vi "Switch Control.vi"(8 "error in (no error)":errorcluster, 11 "On/Off":bool) -> (0 "error out":errorcluster)   [LabVIEW 2014]
doc: "Turns the Switch on or off. Also turns the LED on or off to notify the user which state the switch is in."
uses:
  Controls/Switch Type.ctl
  <vilib>/myRIO/Instrument Drivers/Onboard IO/DIO/vis/Write.vi
  <vilib>/myRIO/Instrument Drivers/Onboard IO/DIO/vis/Smart Open.vi
  <vilib>/Utility/error.llb/Error Cluster From Error Code.vi
  <vilib>/myRIO/Common/Instrument Driver Framework/myRIO v1.0/DIO/vis/myRIO v1.0 Write DIO.vi
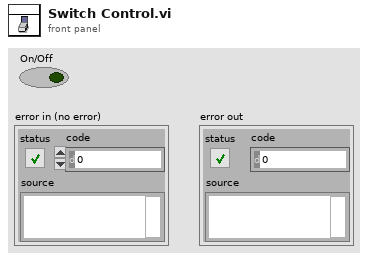
[diagram p1: front panel]
types:
  T1 = typedef "Switch Type.ctl" = enum16{"LED", "Digital Line"}
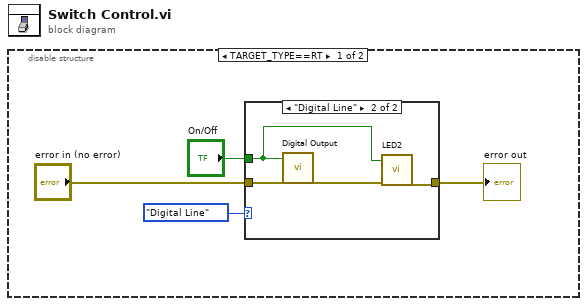
[diagram p0: block diagram]
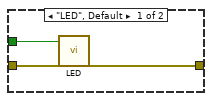
[diagram p2: hidden frame]
diagram:
  n1 = disable-structure shown="TARGET_TYPE==RT" {
    frame condition #0 (active) {
      n2 = case shown="\"Digital Line\"" Switch_Type."Digital Line" {
        tunnel: [w7 w9] -> w4
        tunnel: "error in (no error)" -> [w6 w11]
        tunnel: "On/Off" -> [w5 w8]
        frame "LED", Default {
          n3 = call "LED"("LED0"=w5, "error in (no error)"=w6) -> ("error out"=w7:errorcluster)  [unwired: 25 in]
        }
        frame "Digital Line" {
          n4 = call "Digital Output"("C/DIO7"=w8, "error in (no error)"=w11) -> ("error out"=w10:errorcluster)  [unwired: 25 in]
          n5 = call "LED2"("LED0"=w8, "error in (no error)"=w10) -> ("error out"=w9:errorcluster)  [unwired: 25 in]
        }
      }
      "error out" <- w4
    }
    frame condition #1 {
    }
  }
